vi "HFRR ADV v03.vi"() -> ()   [LabVIEW 2025] (continued)
                n448 = Concatenate Strings("FF ( V ); DP( mincron ) " ("character string"), "\r") -> (w782:string)
                n449 = local read "file count"() -> (w765:i32)
                n450 = local read "FILE 2"() -> (w770:string)
                n451 = local write "save dpt"(FALSE ("Hold 3")) -> ()
                n452 = Number To Decimal String(number=w765) -> (decimal integer string=w771:string)  [unwired: 1 in]
                n453 = Concatenate Strings(w770, w771) -> (w763:string)
                n454 = Concatenate Strings("C:\\LAB-IQ-NXT\\data" ("Substring"), w763) -> (w778:string)
                n455 = Concatenate Strings(w778, ".dpf" ("Substring")) -> (w776:string)
                n456 = Add(x=1, y=w765) -> (x+y=w766:i32)
                n457 = local write "file count"(w766) -> ()
                n458 = String To Path(string=w776) -> (path=w774:path)
                n459 = call <vilib>:"Write Characters To File.vi"("append to file? (new file:F)"=FALSE, "character string"=w782, "file path (dialog if empty)"=w774) -> ("new file path (Not A Path if cancelled)"=w779:path)  [unwired: 2 in]
                n460 = call <vilib>:"Write Characters To File.vi"("append to file? (new file:F)"=TRUE, "character string"=w769, "file path (dialog if empty)"=w779) -> ()  [unwired: 2 in, 1 out]
              }
            }
          }
          frame #5 {
            n461 = case shown="True" "Hold 4" {
              frame False {
              }
              frame True {
                n462 = File Dialog(6:"*.dpf" ("pattern"), 11:path "C:/LAB-IQ-NXT" ("start path")) -> (0:w789:errorcluster, 3:w804:path)  [unwired: 5 in, 2 out]
                n463 = Unbundle(w789) -> ()  [unwired: 3 out]
                n464 = call <vilib>:"Read Characters From File.vi"("file path (dialog if empty)"=w804) -> ("character string"=w794:string)  [unwired: 5 in, 3 out]
                n465 = Spreadsheet String To Array(delimiter (Tab)=";", format string="%S", spreadsheet string=w794, array type (2D Dbl)=string[][] []) -> (array=w798:string[][])
                n466 = for {
                  tunnel: w798 -> [w808] mode=indexing
                  tunnel: [w807] -> w799 mode=indexing
                  n467 = for {
                    tunnel: w808 -> [w810] mode=indexing
                    tunnel: [w809] -> w807 mode=indexing
                    n468 = call <vilib>:"Trim Whitespace.vi"("string"=w810) -> ("trimmed string"=w809:string)  [unwired: 1 in]
                  }
                }
                n469 = Fract/Exp String To Number(string=w799) -> (number=w801:dbl[][])  [unwired: 3 in, 1 out]
                n470 = Array Subset(array=w801, index (row)=1 ("index (col)")) -> (w803:dbl[][])  [unwired: 3 in]
                n471 = Index Array(array=w803, index (col) #1=0 ("disabled index (col)"), index (col) #2=1 ("disabled index (col)")) -> (element #1=w792:dbl[], element #2=w791:dbl[])  [unwired: 2 in]
                n472 = Build Array(w792, w791) -> (→"Waveform Graph":dbl[][])
              }
            }
          }
        }
      }
      frame Error {
        w826 = u16 0 items=["None", "XON/XOFF", "RTS/CTS", "XON/XOFF & RTS/CTS", "DTR/DSR", "XON/XOFF & DTR/DSR"] ("flow control (0:none)  2")
        w824 = u16 10 items=["1.0"=10, "1.5"=15, "2.0"=20] ("stop bits 2")
        w822 = u16 0 items=["None", "Odd", "Even", "Mark", "Space"] ("parity 2")
        w823 = u32 10000  # timeout (10sec)
        n473 = VISA Close(VISA resource name=w818, error in (no error)=w815) -> (error out=w819:errorcluster)
        n474 = local read "Com Port 1"() -> (w811:refnum<visa-resource-name>)
        n475 = call <vilib>:"Clear Errors.vi"("error in (no error)"=w819) -> ("error out"=w816:errorcluster)  [unwired: 5 in, 1 out]
        n476 = local write "Sps 3"(0.0 ("Sps 4")) -> ()
        n477 = call-poly "VISA Configure Serial Port"("VISA resource name"=w811, "timeout (10sec)"=w823, "baud rate (9600)"=u32 250000 ("baud rate  2"), "data bits (8)"=u16 8 ("data bits  2"), "parity (0:none)"=w822, "error in (no error)"=w816, "stop bits (10: 1 bit)"=w824, "flow control (0:none)"=w826) -> ("VISA resource name out"=w827:refnum<visa-resource-name>, "error out"=w828:errorcluster)  [unwired: 6 in]
        n478 = flat-sequence {
          tunnel: w827 -> [w830]
          tunnel: w828 -> [w829]
          tunnel: [w830] -> w820
          tunnel: [w829] -> w812
          frame #0 {
            n479 = Wait (ms)(milliseconds to wait=u32 50) -> ()  [unwired: 1 out]
          }
        }
        "Residual Uno" <- ""
        "Port 1 Error" <- w812
      }
    }
    n480 = local read "Port 1a"() -> (w473:bool)
    n481 = local read "Port 3"() -> (w474:bool)
    n482 = Or(x=w474, y=w473) -> (x .or. y?=w476:bool)
    n483 = case shown="False" w476 {
      frame False {
        w487 = FALSE ("Visible")
        n484 = property on="Port 1a" class="Bool (strict)"("Visible"=w487) -> ()  [unwired: 2 in, 2 out]
        n485 = property on="Port 3" class="Bool (strict)"("Visible"=w487) -> ()  [unwired: 2 in, 2 out]
      }
      frame True {
        w488 = TRUE ("Visible")
        n486 = property on="Port 1a" class="Bool (strict)"("Visible"=w488) -> ()  [unwired: 2 in, 2 out]
        n487 = property on="Port 3" class="Bool (strict)"("Visible"=w488) -> ()  [unwired: 2 in, 2 out]
      }
    }
    n488 = local read "EXIT"() -> (w478:bool)
    "Error Uno" <- w472
  }
  n489 = while {
    tunnel: w54 -> [_]
    tunnel: [w853] -> _
    tunnel: w23 -> [_]
    tunnel: ["EXIT"] -> w51
    i -> [w853]
    stop <- "EXIT" stop-if-true
    # "C:\\LAB-IQ-NXT\\Scar View.exe"
    n490 = local read "RUN"() -> (w851:bool)
    n491 = local read "EDIT 2"() -> (w838:bool)
    n492 = case shown="False" w851 {
      frame False {
        n493 = local read "stopT"() -> (w1724:bool)
        n494 = case shown="True" w1724 {
          frame False {
          }
          frame True {
            w1725 = FALSE
            n495 = local write "st enable"(w1725) -> ()
            n496 = local write "stopT"(w1725) -> ()
          }
        }
      }
      frame True {
        "stopT" <- TRUE
      }
    }
    n497 = case shown="True" w838 {
      frame False {
        n498 = local write "Password 2"("" ("Password")) -> ()
        n499 = property on="Password 2" class="Str"("Visible"=FALSE) -> ()  [unwired: 2 in, 2 out]
      }
      frame True {
        n500 = property on="Password 2" class="Str"("Visible"=TRUE) -> ()  [unwired: 2 in, 2 out]
        n501 = Equal?(x="Password 2", y="HFRR1234") -> (x = y?=w866:bool)
        n502 = case shown="True" w866 {
          tunnel: "Password 2" -> [w869 _]
          frame False {
            n503 = String Length(string=w869) -> (length=w870:i32)
            n504 = Greater Than 0?(x=w870) -> (x > 0?=w868:bool)
            n505 = case shown="False" w868 {
              frame False {
                n506 = property on="Password 2" class="Str"("Caption.Text"="Password (Advance Setting)") -> ()  [unwired: 2 in, 2 out]
              }
              frame True {
                n507 = property on="Password 2" class="Str"("Caption.Text"="Incorrect Password!") -> ()  [unwired: 2 in, 2 out]
              }
            }
          }
          frame True {
            n508 = local write "Password 2"("" ("Password")) -> ()
            n509 = local write "Main Tab"(T1."Advance" ("Main Tab")) -> ()
            n510 = local write "EDIT 2"(FALSE ("EDIT 2")) -> ()
          }
        }
      }
    }
    n511 = Wait (ms)(milliseconds to wait=u32 50) -> ()  [unwired: 1 out]
    n512 = case shown="True" "EDIT 3" {
      frame False {
      }
      frame True {
        n513 = local write "EDIT 3"(FALSE ("EDIT 3")) -> ()
        n514 = local write "Main Tab"(T1."About" ("Main Tab")) -> ()
      }
    }
    n515 = local read "Re-Initialise"() -> (w836:bool)
    n516 = case shown="True" w836 {
      frame False {
      }
      frame True {
        n517 = local write "Re-Initialise"(FALSE ("Re-Initialise")) -> ()
      }
    }
    n518 = case shown="\"ASTM D6079\", Default" "TEST STANDARD" {
      tunnel: [2.0 ("Set Temp") 0.0 ("Set Temp") 2.0 ("Set Temp") 0.0 ("Set Temp")] -> w839
      frame "ASTM D6079", Default {
        # "astm hide"
        n519 = local write "Set Hz"(50.0 ("Hz")) -> ()
        n520 = local write "Set Strk"(1.0 ("Set Strk")) -> ()
        n521 = local write "Set Rh"(53.0 ("Set Rh")) -> ()
        n522 = local write "Set Temp"(60.0 ("Set Temp")) -> ()
        n523 = local write "test time"(75.0 ("test time")) -> ()
        n524 = local write "NORMAL LOAD"(2.0 ("NORMAL LOAD")) -> ()
        "Test Standard" <- "ASTM D6079" ("Test Standard 2")
      }
      frame "ISO 12156" {
        n525 = local write "Set Hz"(50.0 ("Hz")) -> ()
        n526 = local write "Set Rh"(53.0 ("Set Rh")) -> ()
        n527 = local write "Set Strk"(1.0 ("Set Strk")) -> ()
        n528 = local write "test time"(75.0 ("test time")) -> ()
        n529 = local write "Set Temp"(60.0 ("Set Temp")) -> ()
        n530 = local write "NORMAL LOAD"(2.0 ("NORMAL LOAD")) -> ()
      }
      frame "CEC F-096-A-06" {
        n531 = local write "Set Strk"(1.0 ("Set Strk")) -> ()
        n532 = local write "Set Hz"(50.0 ("Hz")) -> ()
        n533 = local write "Set Rh"(53.0 ("Set Rh")) -> ()
        n534 = local write "Set Temp"(60.0 ("Set Temp")) -> ()
        n535 = local write "test time"(75.0 ("test time")) -> ()
        n536 = local write "NORMAL LOAD"(2.0 ("NORMAL LOAD")) -> ()
      }
      frame "Custom" {
      }
    }
    n537 = local read "OPEN 6"() -> (w835:bool)
    n538 = local read "service 3"() -> (w833:bool)
    n539 = Or(x=w835, y=w833) -> (x .or. y?=w834:bool)
    n540 = local read "RUN"() -> (w848:bool)
    n541 = case shown="True" w834 {
      selector: w834 -> [_ w858]
      frame False {
      }
      frame True {
        n542 = Not(x=w858) -> (.not. x?=w854:bool)
        n543 = local write "service 3"(w854) -> ()
        n544 = local write "OPEN 6"(w854) -> ()
        n545 = call <vilib>:"System Exec.vi"("wait until completion? (T)"=TRUE, "command line"="C:\\LAB-IQ-NXT\\Scar View.exe") -> ("error out"=→"error out 5":errorcluster)  [unwired: 6 in, 3 out]
      }
    }
    n546 = case shown="True" w848 {
      frame False {
      }
      frame True {
        n547 = local read "Main Tab"() -> (w1722:T1)
        n548 = case shown="\"Compare Files\"" w1722 {
          frame "Acquire", Default {
          }
          frame "Compare Files" {
            n549 = local write "Main Tab"(T1."Acquire" ("Main Tab")) -> ()
          }
          frame "About" {
          }
        }
      }
    }
    n550 = local read "Main Tab"() -> (w832:T1)
    n551 = case shown="\"Compare Files\"" w832 {
      tunnel: [T12."Acquire" ("Main Tab") T13."   COMPARE   FILES " ("Tab Control") T14."PRINT REPORT" ("Tab Control")] -> w846
      frame "Acquire", Default {
      }
      frame "Compare Files" {
      }
      frame "About" {
      }
    }
    n552 = property on="SetTemp" class="DigNum (strict)"("Disabled"=w839) -> ()  [unwired: 2 in, 2 out]
    n553 = case shown="0, Default" w846 {
      frame 0, Default {
        w1866 = 0.2 ("y")
        w1871 = 1.0 ("y")
        w1872 = 0.8 ("y")
        # "Elapsed time\ncof\nstroke\nAir temp\nTemp\nHumidity"
        n554 = case shown="True" "Save & Continue" {
          frame False {
          }
          frame True {
            "acq 2" <- TRUE ("acq 2")
          }
        }
        n555 = case shown="True" "Save & Continue" {
          frame False {
          }
          frame True {
            n556 = while {
              tunnel: "0123456789abcdefghijklmnopqrstuvwxyzABCDEFGHIJKLMNOPQRSTUVWXYZ" ("string 2") -> [w1990]
              shift-right: [w1988] -> w1983
              shift-left: "" -> [w1987]
              i -> [w1997]
              stop <- w1996 stop-if-true
              n557 = Random Number (0-1)() -> (number: 0 to 1=w1991:dbl)
              n558 = Multiply(x=w1991, y=62.0) -> (x*y=w1993:dbl)
              n559 = Decrement(x="Length") -> (x-1=w1986:i16)
              n560 = To Word Integer(number=w1993) -> (16bit integer=w1994:i16)
              n561 = String Subset(string=w1990, offset (0)=w1994, length (rest)=1 ("length (rest)")) -> (substring=w1989:string)
              n562 = Greater Or Equal?(x=w1997, y=w1986) -> (x >= y?=w1996:bool)
              n563 = Concatenate Strings(w1989, w1987) -> (w1988:string)
            }
            n564 = local write "UUID"(w1983) -> ()
          }
        }
        n565 = case shown="True" "Save & Continue" {
          frame False {
          }
          frame True {
            n566 = local read "Operator ID"() -> (w2273:string)
            n567 = local read "FILE"() -> (w2280:string)
            n568 = String Length(string=w2273) -> (length=w2274:i32)
            n569 = String Length(string=w2280) -> (length=w2278:i32)
            n570 = Greater?(x=w2274, y=0) -> (0:w2272:bool)
            n571 = Greater?(x=w2278, y=0) -> (0:w2277:bool)
            n572 = And(x=w2277, y=w2272) -> (x .and. y?=w2276:bool)
            n573 = case shown="True" w2276 {
              frame False {
                n574 = stacked-sequence {
                  frame #0 {
                    n575 = One Button Dialog(message="Please Enter a File Name and Operator ID to save data !", button name ("OK")="Ok") -> ()  [unwired: 1 out]
                  }
                  frame #1 {
                    n576 = local write "Save & Continue"(FALSE ("OK Button")) -> ()
                  }
                }
                n577 = local write "Save & Continue"(FALSE ("OK Button")) -> ()
              }
              frame True {
                n578 = stacked-sequence {
                  frame #0 {
                    (unwired) ")!" ("string")
                    (unwired) ")" ("string")
                    w2285 = dbl[] [] ("History Data")
                    w2289 = "\r"
                    # "C:\\WinDucom\\Data\\"
                    # "C:\\LAB-IQ-NXT\\data"
                    n579 = local read "Batch Ref Num :"() -> (w2287:string)
                    n580 = local read "NORMAL LOAD"() -> (w2306:dbl)
                    n581 = local read "Fuel Discription :"() -> (w2300:string)
                    n582 = Multiply(x=w2306, y=1.0) -> (x*y=w2305:dbl)
                    n583 = Number To Fractional String(number=w2305, width (-)=i16 5, precision (6)=i16 2) -> (F-format string=w2314:string)  [unwired: 1 in]
                    n584 = Concatenate Strings(w2300) -> (w2301:string)
                    n585 = local read "Remarks :"() -> (w2299:string)
                    n586 = property on="Electronic contact resistance ( % )" class="WFChart (strict)"("History Data"=w2285) -> ()  [unwired: 2 in, 2 out]
                    n587 = Get Date/Time String(date format (0)=enum16{"short", "long", "abbreviated"}."short") -> (date string=w2325:string, time string=w2322:string)  [unwired: 2 in]
                    n588 = property on="Coefficient of Friction" class="WFChart (strict)"("History Data"=w2285) -> ()  [unwired: 2 in, 2 out]
                    n589 = property on="Frictional Force ( N )" class="WFChart (strict)"("History Data"=w2285) -> ()  [unwired: 2 in, 2 out]
                    n590 = Concatenate Strings(w2287) -> (w2286:string)
                    n591 = Concatenate Strings(w2299, "," ("string")) -> (w2298:string)
                    n592 = Concatenate Strings("Load :- " ("Substring"), w2314, " N ," ("Substring")) -> (w2313:string)
                    n593 = local read "String 41"() -> (w2291:string)
                    n594 = local read "FILE"() -> (w2333:string)
                    n595 = Concatenate Strings("(" ("Substring"), w2325, ")" ("Substring"), w2322) -> (w2293:string)
                    "concatenated string" <- w2293
                    n596 = Concatenate Strings("C:\\LAB-IQ-NXT\\data\\" ("string"), w2333) -> (w2332:string)
                    n597 = Concatenate Strings("tested by") -> (w2295:string)
                    n598 = Concatenate Strings(w2332, ".duf" ("Substring")) -> (w2329:string)
                    n599 = Concatenate Strings(w2332, ".dgf" ("Substring")) -> (w2328:string)
                    n600 = String To Path(string=w2328) -> (path=w2326:path)
                    n601 = String To Path(string=w2329) -> (path=w2303:path)
                    n602 = Concatenate Strings(w2291, w2289, "Fuel Discription :-" ("Substring"), w2301, w2289, w2313, w2289, "Batch Ref Num :-" ("Substring"), w2286, w2289, " Remarks :- " ("Substring"), w2298, w2289, " Date :- " ("Substring"), w2293, w2289, "Tested By :-" ("Substring"), w2295) -> (w2307:string)
                    "REMARKS" <- w2307
                    n603 = local write "clk"(0.0 ("clk")) -> ()
                    n604 = local write "speedop"(0.0 ("PIDclk 2")) -> ()
                    n605 = Concatenate Strings("  TIME;      COF;       STROKE;     AIR TEMP;  TEMP;  HUMIDITY;  ECR; PID-OUT; FREQUENCY" ("Substring"), "\r") -> (w2309:string)
                    n606 = call <vilib>:"Write Characters To File.vi"("append to file? (new file:F)"=FALSE, "character string"=w2309, "file path (dialog if empty)"=w2326) -> ()  [unwired: 2 in, 1 out]
                    n607 = call <vilib>:"Write Characters To File.vi"("append to file? (new file:F)"=FALSE, "character string"=w2307, "file path (dialog if empty)"=w2303) -> ()  [unwired: 2 in, 1 out]
                  }
                  frame #1 {
                    n608 = local write "autostrtflg"(TRUE ("autostrtflg")) -> ()
                    n609 = local write "Save & Continue"(FALSE ("OK")) -> ()
                    n610 = local write "STOP 3"(FALSE ("STOP")) -> ()
                    n611 = One Button Dialog(message="Please ensure sample is mounted properly and machine is ready in all aspects for testing !", button name ("OK")="Ok") -> ()  [unwired: 1 out]
                    n612 = property on="Save & Continue" class="Bool (strict)"("Visible"=FALSE ("OK")) -> ()  [unwired: 2 in, 2 out]
                    n613 = property on="STOP 3" class="Bool (strict)"("Visible"=TRUE) -> ()  [unwired: 2 in, 2 out]
                    n614 = Get Date/Time In Seconds() -> (seconds since 1Jan1904=w2338:timestamp)
                    n615 = local write "Cycles elapsed"(0 ("Cycles elapsed")) -> ()
                    n616 = To Double Precision Float(number=w2338) -> (double precision float=w2337:dbl)
                    n617 = local write "cyclecount"(0 ("cyclecount")) -> ()
                    n618 = local write "acq timer"(w2337) -> ()
                    n619 = local write "Save"(FALSE ("Save")) -> ()
                  }
                }
              }
            }
          }
        }
        n620 = case shown="True" "Case Constant\n(See Context Help) 15" {
          frame False {
          }
          frame True {
            n621 = local read "zflag 2"() -> (w1898:dbl)
            n622 = local read "yflag"() -> (w1900:dbl)
            n623 = Equal?(x=w1898, y=3.0 ("tflag")) -> (x = y?=w1901:bool)
            n624 = Equal?(x=w1900, y=2.0 ("tflag")) -> (x = y?=w1902:bool)
            n625 = And(x=w1902, y=w1901) -> (x .and. y?=w1896:bool)
            n626 = case shown="True" w1896 {
              frame False {
              }
              frame True {
                w1927 = 0.0 ("zflag")
                n627 = local read "SEN.RUN HRS"() -> (w1913:dbl)
                n628 = local read "SENSOR TIME"() -> (w1911:dbl)
                n629 = local read "Total No. of Tests"() -> (w1914:dbl)
                n630 = Delete(path (use dialog)=path "C:/LAB-IQ-NXT/WO 2449 TRH.sig" ("file path (dialog if empty)")) -> (deleted path=w1921:path)  [unwired: 4 in, 2 out]
                n631 = Add(x=w1911, y=w1913) -> (x+y=w1912:dbl)
                "SEN.RUN HRS" <- w1912
                n632 = Number To Decimal String(number=w1912) -> (decimal integer string=w1918:string)  [unwired: 1 in]
                n633 = call <vilib>:"compatOverwrite.vi"("overwrite (F)"=TRUE) -> ("overwrite?"=w1907:T17)
                n634 = Delete(path (use dialog)=path "C:/LAB-IQ-NXT/WO 2449 TT.sig" ("file path (dialog if empty)")) -> (deleted path=w1926:path)  [unwired: 4 in, 2 out]
                n635 = Open/Create/Replace File(file path (use dialog)=w1921, operation (0:open)=w1907) -> (refnum out=w1908:refnum<file>, error out=w1909:errorcluster)  [unwired: 4 in, 1 out]
                n636 = Number To Decimal String(number=w1914) -> (decimal integer string=w1922:string)  [unwired: 1 in]
                n637 = Deny Access(4:w1909, 6:T15."deny none" ("deny mode (2)"), 7:w1908) -> (3:w1917:refnum<file>)  [unwired: 1 out]
                n638 = call <vilib>:"compatOverwrite.vi"("overwrite (F)"=TRUE) -> ("overwrite?"=w1903:T17)
                n639 = Write to Binary File(file (use dialog)=w1917, data=w1918, 5:FALSE ("prepend array or string size? (T)")) -> ()  [unwired: 3 in, 3 out]
                n640 = Open/Create/Replace File(file path (use dialog)=w1926, operation (0:open)=w1903) -> (refnum out=w1904:refnum<file>, error out=w1905:errorcluster)  [unwired: 4 in, 1 out]
                n641 = Deny Access(4:w1905, 6:T15."deny none" ("deny mode (2)"), 7:w1904) -> (3:w1925:refnum<file>)  [unwired: 1 out]
                n642 = local write "zflag"(w1927) -> ()
                n643 = local write "zflag 2"(w1927) -> ()
                n644 = Write to Binary File(file (use dialog)=w1925, data=w1922, 5:FALSE ("prepend array or string size? (T)")) -> ()  [unwired: 3 in, 3 out]
              }
            }
          }
        }
        n645 = case shown="True" "STOP 3" {
          frame False {
          }
          frame True {
            w2265 = "" ("Sample ID :")
            (unwired) FALSE ("Visible")
            n646 = local write "Save & Continue"(FALSE ("OK Button")) -> ()
            n647 = local write "STOP 3"(FALSE ("STOP")) -> ()
            n648 = local write "clk"(0.0 ("clk")) -> ()
            n649 = local write "RUN"(FALSE ("OK Button 2")) -> ()
            n650 = property on="Save & Continue" class="Bool (strict)"("Visible"=TRUE) -> ()  [unwired: 2 in, 2 out]
            n651 = property on="STOP 3" class="Bool (strict)"("Visible"=FALSE) -> ()  [unwired: 2 in, 2 out]
            n652 = property on="STOP 2" class="Bool (strict)"("Disabled"=u8 0) -> ()  [unwired: 2 in, 2 out]
            n653 = local write "Fuel Discription :"(w2265) -> ()
            n654 = local write "Remarks :"(w2265) -> ()
            n655 = local write "tested by"(w2265) -> ()
            n656 = local write "FILE"(w2265) -> ()
            n657 = local write "Batch Ref Num :"(w2265) -> ()
          }
        }
        n658 = local read "AIR TEMP"() -> (w1838:dbl)
        n659 = local read "run replace"() -> (w1878:bool)
        n660 = Greater Or Equal?(x=w1838, y=15.0) -> (x >= y?=w1839:bool)
        "powstat" <- w1839
        n661 = local read "acq 2"() -> (w1877:bool)
        n662 = And(x=w1877, y=w1878) -> (x .and. y?=w1876:bool)
        n663 = local read "run replace"() -> (w1879:bool)
        n664 = case shown="True" w1876 {
          frame False {
            n665 = local write "tfalg"(0.0 ("tfalg")) -> ()
          }
          frame True {
            n666 = local read "tfalg"() -> (w1974:dbl)
            n667 = Equal?(x=w1974, y=0.0) -> (x = y?=w1975:bool)
            n668 = case shown="True" w1975 {
              frame False {
              }
              frame True {
                n669 = local read "Total No. of Tests"() -> (w1978:dbl)
                n670 = Increment(x=w1978) -> (x+1=w1977:dbl)
                n671 = local write "Total No. of Tests"(w1977) -> ()
                n672 = local write "tfalg"(1.0 ("tfalg")) -> ()
                n673 = local write "acq 2"(FALSE ("acq 2")) -> ()
                n674 = Wait (ms)(milliseconds to wait=u32 200) -> ()  [unwired: 1 out]
              }
            }
          }
        }
        n675 = case shown="False" w1879 {
          frame False {
            n676 = local read "zflag"() -> (→"zflag 2":dbl)
            n677 = local write "FLAG 4"(0.0 ("FLAG")) -> ()
            n678 = local write "yflag"(2.0 ("tflag")) -> ()
          }
          frame True {
            n679 = local write "zflag"(3.0 ("zflag")) -> ()
            n680 = local write "yflag"(1.0 ("tflag")) -> ()
          }
        }
        n681 = property on="STOP 3" class="Bool (strict)"() -> ("Visible"=w1881:bool)  [unwired: 2 in, 2 out]
        n682 = case shown="True" w1881 {
          tunnel: [FALSE ("Visible") TRUE ("Visible")] -> w1891
          frame False {
          }
          frame True {
          }
        }
        n683 = property on="RUN" class="Bool (strict)"("Visible"=w1891) -> ()  [unwired: 2 in, 2 out]
        n684 = property on="Save & Continue" class="Bool (strict)"() -> ("Visible"=w1894:bool)  [unwired: 2 in, 2 out]
        n685 = local read "RUN"() -> (w1875:bool)
        n686 = case shown="True" w1875 {
          frame False {
            n687 = local read "Rt 3"() -> (w1956:bool)
            n688 = case shown="True" w1956 {
              frame False {
              }
              frame True {
                n689 = local write "Json End Flg"(TRUE ("Upld AR 2")) -> ()
                n690 = local write "Rt 3"(FALSE ("Rt 3")) -> ()
              }
            }
            "Rt" <- TRUE ("Rt")
            "Rt 2" <- FALSE ("Rt")
          }
          frame True {
            n691 = local read "Rt"() -> (w1963:bool)
            n692 = case shown="True" w1963 {
              frame False {
              }
              frame True {
                w1964 = TRUE ("Upld AR 2")
                n693 = local write "Rt"(FALSE ("Rt")) -> ()
                n694 = local write "Upld AR"(w1964) -> ()
                n695 = local write "Json St Flg"(w1964) -> ()
              }
            }
            n696 = local write "Rt 2"(TRUE ("Rt 2")) -> ()
            "Rt 3" <- TRUE ("Rt 3")
          }
        }
        n697 = Not(x=w1894) -> (.not. x?=w1893:bool)
        n698 = case shown="True" w1875 {
          frame False {
            n699 = local write "run replace"(FALSE ("run replace")) -> ()
          }
          frame True {
            "run replace" <- TRUE ("run replace")
          }
        }
        n700 = And(x=w1893, y=w1881) -> (x .and. y?=w1890:bool)
        "Test Status 2" <- w1890
        n701 = case shown="True" w1890 {
          tunnel: w1839 -> [_ w2029]
          frame False {
            w2027 = 0.0 ("output")
            n702 = local write "Frequency ( Hz )"(w2027) -> ()
            n703 = local write "PID-out"(w2027) -> ()
            n704 = local write "Heater Button"(FALSE ("Heater Button")) -> ()
          }
          frame True {
            n705 = case shown="False" w2029 {
              frame False {
                n706 = stacked-sequence {
                  frame #0 {
                    n707 = local write "RUN"(FALSE ("OK Button 2")) -> ()
                  }
                  frame #1 {
                    n708 = property on="RUN" class="Bool (strict)"("Visible"=FALSE) -> ()  [unwired: 2 in, 2 out]
                  }
                }
              }
              frame True {
              }
            }
            n709 = stacked-sequence {
              frame #0 {
                n710 = case shown="True" "RUN" {
                  tunnel: [w2056 w2064] -> w2033
                  frame False {
                    w2056 = 0.0
                    n711 = local write "Reinit PID"(TRUE) -> ()
                    n712 = property on="Stroke 2" class="DigNum (strict)"("Visible"=FALSE) -> ()  [unwired: 2 in, 2 out]
                    n713 = property on="Stroke" class="DigNum (strict)"("Visible"=TRUE) -> ()  [unwired: 2 in, 2 out]
                    n714 = local write "String 14"("Test will autostart once parameters reach the set value." ("String 14")) -> ()
                    n715 = local write "Old Pid Val"(w2056) -> ()
                  }
                  frame True {
                    n716 = local read "PID Ref"() -> (w2075:bool)
                    n717 = property on="STOP 2" class="Bool (strict)"("Disabled"=u8 2) -> ()  [unwired: 2 in, 2 out]
                    n718 = case shown="True" w2075 {
                      tunnel: [w2076 w2092] -> w2074
                      frame False {
                        n719 = local read "Old Pid Val"() -> (w2076:dbl)
                      }
                      frame True {
                        n720 = local read "Set Hz"() -> (w2085:dbl)
                        n721 = Add(x=w2085, y=-10.0 ("Offset")) -> (x+y=w2103:dbl)
                        n722 = local read "Frequency"() -> (w2096:dbl)
                        n723 = Add(x=w2085, y=-10.0) -> (x+y=w2095:dbl)
                        n724 = Add(x=w2085, y=10.0) -> (x+y=w2094:dbl)
                        n725 = Multiply(x=w2103, y=0.1 ("Gain")) -> (x*y=w2082:dbl)
                        n726 = Add(x=w2082, y=1.5) -> (x+y=w2080:dbl)
                        n727 = local read "SPEED OUT:"() -> (w2104:dbl)
                        n728 = In Range and Coerce(upper limit=w2094, x=w2096, lower limit=w2095) -> (coerced(x)=w2084:dbl)  [unwired: 1 out]
                        n729 = Multiply(x=w2080, y=w2104) -> (x*y=w2079:dbl)
                        n730 = Multiply(x=w2079, y=0.8) -> (x*y=w2078:dbl)
                        n731 = local read "Elapsed time"() -> (w2089:dbl)
                        n732 = Or(x="Reinit PID", y="Reinit PID") -> (x .or. y?=w2093:bool)
                        n733 = call-poly <vilib>:"PID.vi"("reinitialize? (F)"=w2093, "output range"=cluster{"output high":dbl, "output low":dbl} {"output high"=1.0, "output low"=-1.0}, "PID gains"=T7 {"proportional gain (Kc)"=0.0005, "integral time (Ti, min)"=0.001, "derivative time (Td, min)"=0.0} ("Motor PID"), "process variable"=w2084, "setpoint"=w2085) -> ("output"=w2083:dbl)  [unwired: 5 in, 1 out]
                        n734 = Greater?(x=w2089, y=0.05) -> (0:w2088:bool)
                        n735 = case shown="True" w2088 {
                          tunnel: w2083 -> [_ w2106]
                          tunnel: [0.0 ("output") w2106] -> w2086
                          frame False {
                          }
                          frame True {
                            n736 = local write "Reinit PID"(FALSE ("Reinit PID")) -> ()
                          }
                        }
                        n737 = Add(x=w2078, y=w2086) -> (x+y=w2091:dbl)
                        n738 = flat-sequence {
                          tunnel: [w2109] -> w2092
                          tunnel: w2091 -> [w2109]
                          frame #0 {
                            n739 = local write "PID Ref"(FALSE ("PID Ref")) -> ()
                          }
                        }
                      }
                    }
                    "Old Pid Val" <- w2074
                    n740 = local read "Set Hz"() -> (w2071:dbl)
                    n741 = local read "Freq"() -> (w2063:dbl)
                    n742 = call <vilib>:"Uniform White Noise Waveform.vi"() -> ("signal out"=w2070:waveform(dbl))  [unwired: 10 in, 1 out]
                    n743 = property on="RUN" class="Bool (strict)"("Visible"=TRUE) -> ()  [unwired: 2 in, 2 out]
                    n744 = Add(x=w2071, y=w2070) -> (x+y=w2069:waveform(dbl))
                    n745 = property on="Stroke 2" class="DigNum (strict)"("Visible"=TRUE) -> ()  [unwired: 2 in, 2 out]
                    n746 = property on="Stroke" class="DigNum (strict)"("Visible"=FALSE) -> ()  [unwired: 2 in, 2 out]
                    n747 = Multiply(x=w2069, y=ext 0.1) -> (x*y=w2065:waveform(ext))
                    n748 = Multiply(x=w2063, y=0.9) -> (x*y=w2066:dbl)
                    n749 = local write "String 14"(" Running....." ("String 14")) -> ()
                    n750 = Add(x=w2065, y=w2066) -> (x+y=w2064:waveform(ext))
                  }
                }
                n751 = Not(x="Engage") -> (.not. x?=w2037:bool)
                n752 = call "Elapsed Time"("Time Target (s)"="Countdown", "Reset"=w2037) -> ("Elapsed Time (s)"=w2042:dbl, "Time has Elapsed"=w2040:bool)  [unwired: 10 in, 6 out]
                "Countdown 2" <- w2042
                n753 = Subtract(x=w2042, y=2.0) -> (x-y=w2045:dbl)
                n754 = Less?(x=w2045, y="Countdown") -> (x < y?=w2043:bool)
                n755 = And(x=w2043, y=w2040) -> (x .and. y?=w2039:bool)
                n756 = case shown="True" w2039 {
                  frame False {
                  }
                  frame True {
                    n757 = local read "Humidity ( Rh )"() -> (→"Rh Before":dbl)
                    n758 = local write "RUN"(TRUE ("RUN")) -> ()
                    n759 = local write "Engage"(FALSE ("Engage")) -> ()
                    n760 = property on="gRh" class="WFChart (strict)"("History Data"=dbl[] []) -> ()  [unwired: 2 in, 2 out]
                  }
                }
                n761 = local read "clk"() -> (w2050:dbl)
                n762 = local read "Save"() -> (w2046:bool)
                n763 = Equal?(x=w2050, y=0.0) -> (x = y?=w2047:bool)
                n764 = And(x=w2047, y=w2046) -> (x .and. y?=w2048:bool)
                n765 = case shown="True" w2048 {
                  frame False {
                  }
                  frame True {
                    n766 = Get Date/Time In Seconds() -> (seconds since 1Jan1904=w2112:timestamp)
                    n767 = To Double Precision Float(number=w2112) -> (double precision float=w2110:dbl)
                    n768 = local write "act save time"(w2110) -> ()
                    n769 = local write "acq timer"(w2110) -> ()
                    n770 = local write "clk"(10.0 ("clk")) -> ()
                  }
                }
                n771 = local read "Test \nStatus"() -> (w2035:bool)
                n772 = Select(t=w2033, s=w2035, f=0.0) -> (s? t:f=w2034:dbl)
                n773 = local write "Frequency ( Hz )"(w2034) -> ()
                n774 = local write "Freq"(w2034) -> ()
              }
              frame #1 {
                w2135 = 1000000.0 ("x")
                # "Elapsed time\ncof\nstroke\nAir temp\nTemp\nHumidity"
                # "acq timer\n\nact save time"
                # "convert to microseconds"
                n775 = local read "COUNT"() -> (w2118:i32)
                n776 = Greater Or Equal?(x=w2118, y=250) -> (x >= y?=w2117:bool)
                n777 = case shown="True" w2117 {
                  frame False {
                    n778 = local read "COUNT"() -> (w2139:i32)
                    n779 = Increment(x=w2139) -> (x+1=w2140:i32)
                    n780 = local write "COUNT"(w2140) -> ()
                  }
                  frame True {
                    n781 = local write "COUNT"(0 ("COUNT")) -> ()
                  }
                }
                n782 = local read "Samplingtime 2"() -> (w2116:dbl)
                n783 = local read "act save time"() -> (w2133:dbl)
                n784 = Get Date/Time In Seconds() -> (seconds since 1Jan1904=w2138:timestamp)
                n785 = To Double Precision Float(number=w2138) -> (double precision float=w2127:dbl)
                n786 = local read "acq timer"() -> (w2137:dbl)
                n787 = Add(x=w2133, y=w2116) -> (x+y=w2132:dbl)
                n788 = Greater Or Equal?(x=w2127, y=w2132) -> (x >= y?=w2115:bool)
                n789 = Subtract(x=w2127, y=w2137) -> (x-y=w2129:dbl)
                n790 = local read "Rate"() -> (w2131:dbl)
                n791 = Divide(x=w2135, y=w2131) -> (x/y=w2136:dbl)
                n792 = Divide(x=w2136, y=w2135) -> (x/y=w2134:dbl)
                n793 = local read "Save"() -> (w2130:bool)
                n794 = And(x=w2115, y=w2130) -> (x .and. y?=w2128:bool)
                n795 = case shown="True" w2128 {
                  tunnel: w2127 -> [_ w2210]
                  tunnel: [FALSE ("Boolean 2") TRUE ("Boolean 2")] -> _
                  frame False {
                  }
                  frame True {
                    w2178 = ";" ("Substring")
                    # "Pid out/\nFreq response value"
                    n796 = local write "act save time"(w2210) -> ()
                    n797 = local read "Set Strk"() -> (w2177:dbl)
                    n798 = local read "Stroke"() -> (w2167:dbl)
                    n799 = local read "FF 2"() -> (w2163:dbl)
                    "Frictional Force ( N )" <- w2163
                    n800 = Subtract(x=w2167, y=w2177) -> (x-y=w2174:dbl)
                    n801 = local read "TEMP"() -> (w2164:dbl)
                    "Temp" <- w2164
                    n802 = local write "FF 3"(w2163) -> ()
                    n803 = local read "ecr"() -> (w2162:dbl)
                    "ecr 2" <- w2162
                    n804 = Multiply(x=w2174, y=0.05) -> (x*y=w2176:dbl)
                    n805 = local read "Humidity ( Rh )"() -> (w2185:dbl)
                    "gRh" <- w2185
                    n806 = local read "Frequency ( Hz )"() -> (w2170:dbl)
                    n807 = local write "ecr 3"(w2162) -> ()
                    n808 = local read "COF 2"() -> (w2165:dbl)
                    "cof" <- w2165
                    "Coefficient of Friction" <- w2165
                    n809 = Add(x=w2176, y=w2177) -> (x+y=w2168:dbl)
                    "Stroke Ln" <- w2168
                    "Stroke 2" <- w2168
                    "Disp" <- w2168
                    n810 = local write "Temperature ( Deg C )"(w2164) -> ()
                    n811 = local read "Elapsed time"() -> (w2203:dbl)
                    n812 = local write "COF 3"(w2165) -> ()
                    n813 = local read "AIR TEMP"() -> (w2166:dbl)
                    n814 = local write "Electronic contact resistance ( % )"(w2162) -> ()
                    n815 = local read "PID-out"() -> (w2173:dbl)
                    n816 = local read "FILE"() -> (w2211:string)
                    n817 = Number To Fractional String(number=w2165, width (-)=i16 9 ("precision (6)"), precision (6)=i16 6) -> (F-format string=w2204:string)  [unwired: 1 in]
                    n818 = Number To Fractional String(number=w2168, width (-)=i16 9 ("precision (6)"), precision (6)=i16 6) -> (F-format string=w2196:string)  [unwired: 1 in]
                    n819 = Number To Fractional String(number=w2166, width (-)=i16 9 ("precision (6)"), precision (6)=i16 3) -> (F-format string=w2195:string)  [unwired: 1 in]
                    n820 = Number To Fractional String(number=w2164, width (-)=i16 9 ("precision (6)"), precision (6)=i16 3) -> (F-format string=w2192:string)  [unwired: 1 in]
                    n821 = Number To Fractional String(number=w2185, width (-)=i16 9 ("precision (6)"), precision (6)=i16 3) -> (F-format string=w2189:string)  [unwired: 1 in]
                    n822 = Number To Fractional String(number=w2162, width (-)=i16 9 ("precision (6)"), precision (6)=i16 3) -> (F-format string=w2184:string)  [unwired: 1 in]
                    n823 = Number To Fractional String(number=w2173, width (-)=i16 9 ("precision (6)"), precision (6)=i16 3) -> (F-format string=w2179:string)  [unwired: 1 in]
                    n824 = Number To Fractional String(number=w2170, width (-)=i16 9 ("precision (6)"), precision (6)=i16 3) -> (F-format string=w2169:string)  [unwired: 1 in]
                    n825 = Number To Fractional String(number=w2203, width (-)=i16 14 ("precision (6)"), precision (6)=i16 3) -> (F-format string=w2205:string)  [unwired: 1 in]
                    n826 = Concatenate Strings("C:\\LAB-IQ-NXT\\Data\\" ("string"), w2211, ".dgf" ("Substring")) -> (w2213:string)
                    n827 = String To Path(string=w2213) -> (path=w2212:path)
                    n828 = Concatenate Strings(w2205, w2178, w2204, w2178, w2196, w2178, w2195, w2178, w2192, w2178, w2189, w2178, w2184, w2178, w2179, w2178, w2169, "\r") -> (w2202:string)
                    n829 = call <vilib>:"Write Characters To File.vi"("append to file? (new file:F)"=TRUE, "character string"=w2202, "file path (dialog if empty)"=w2212) -> ()  [unwired: 2 in, 1 out]
                    "refresh flag" <- TRUE ("refresh flag")
                  }
                }
                n830 = local read "COUNT"() -> (w2120:i32)
                n831 = Multiply(x=w2134, y=w2120) -> (x*y=w2126:dbl)
                n832 = Add(x=w2129, y=w2126) -> (x+y=w2113:dbl)
                "Elapsed time 3" <- w2113
                n833 = local read "Test \nStatus"() -> (w2114:bool)
                n834 = local read "clk"() -> (w2121:dbl)
                n835 = Equal?(x=w2121, y=10.0) -> (x = y?=w2123:bool)
                n836 = Divide(x=w2113, y=60.0) -> (x/y=w2124:dbl)
                n837 = case shown="True" w2114 {
                  tunnel: w2124 -> [_ w2146]
                  tunnel: w2129 -> [_ w2154]
                  tunnel: [0.0 w2150] -> _
                  tunnel: w2123 -> [_ w2149]
                  tunnel: [0.0 w2148] -> _
                  tunnel: w2113 -> [_ w2148]
                  tunnel: w2127 -> [w2142 _]
                  frame False {
                    n838 = local write "acq timer"(w2142) -> ()
                  }
                  frame True {
                    n839 = local read "Set Hz"() -> (w2151:dbl)
                    n840 = local write "Elapsed time"(w2146) -> ()
                    n841 = local read "test time"() -> (w2147:dbl)
                    n842 = Multiply(x=w2154, y=w2151) -> (x*y=w2153:dbl)
                    n843 = case shown="False" w2149 {
                      tunnel: w2153 -> [w2155 _]
                      tunnel: [w2155 1.0] -> w2150
                      frame False {
                        n844 = local write "Cycles elapsed"(w2155) -> ()
                      }
                      frame True {
                      }
                    }
                    n845 = Subtract(x=w2147, y=w2146) -> (x-y=w2145:dbl)
                    "time" <- w2145
                    n846 = Greater?(x=w2146, y=w2147) -> (0:w2152:bool)
                    n847 = case shown="True" w2152 {
                      frame False {
                      }
                      frame True {
                        n848 = local read "Humidity ( Rh )"() -> (→"Rh After":dbl)
                        n849 = property on="STOP 2" class="Bool (strict)"("Disabled"=u8 0) -> ()  [unwired: 2 in, 2 out]
                        n850 = local write "RUN"(FALSE ("OK Button 2")) -> ()
                        n851 = local write "STOP 3"(TRUE ("STOP")) -> ()
                      }
                    }
                    n852 = local write "Time Remaining"(w2145) -> ()
                  }
                }
              }
              frame #2 {
                n853 = case shown="True" "Heater Button" {
                  tunnel: [0.0 ("output") w2237] -> w2216
                  frame False {
                    w2218 = TRUE ("tmpchk")
                    n854 = local write "tmpchk"(w2218) -> ()
                    n855 = local write "Reset 4"(w2218) -> ()
                    n856 = local read "TEMP"() -> (w2219:dbl)
                    n857 = local write "Temp ini"(w2219) -> ()
                    n858 = local write "reinit"(TRUE ("reinit")) -> ()
                  }
                  frame True {
                    # "Logic to turn off\nthe heater when \ntemp is not rising.\nTime - 60 sec\nDelta t- 5°c"
                    n859 = local read "Set Temp"() -> (w2234:dbl)
                    n860 = local read "Temp ini"() -> (w2225:dbl)
                    n861 = local read "TEMP"() -> (w2228:dbl)
                    n862 = Add(x=w2234, y=0.5) -> (x+y=w2232:dbl)
                    n863 = Less?(x=w2225, y=53.0) -> (x < y?=w2223:bool)
                    n864 = Greater Or Equal?(x=w2228, y=w2232) -> ()  [unwired: 1 out]
                    n865 = And(x="tmpchk", y=w2223) -> (x .and. y?=w2226:bool)
                    n866 = case shown="True" w2226 {
                      frame False {
                      }
                      frame True {
                        n867 = call "Elapsed Time8"("Time Target (s)"=300.0, "Reset"="Reset 4") -> ("Time has Elapsed"=w2242:bool)  [unwired: 10 in, 7 out]
                        n868 = flat-sequence {
                          tunnel: w2242 -> [_]
                          frame #0 {
                            n869 = local write "Reset 4"(FALSE ("Reset 4")) -> ()
                          }
                        }
                        n870 = case shown="True" w2242 {
                          frame False {
                          }
                          frame True {
                            n871 = local read "Temp ini"() -> (w2249:dbl)
                            n872 = local read "TEMP"() -> (w2250:dbl)
                            n873 = Add(x=w2249, y=5.0) -> (x+y=w2247:dbl)
                            n874 = Greater?(x=w2250, y=w2247) -> (0:w2248:bool)
                            n875 = case shown="False" w2248 {
                              frame False {
                                n876 = local write "Heater Button"(FALSE ("Heater Button")) -> ()
                              }
                              frame True {
                                n877 = local write "tmpchk"(FALSE ("tmpchk")) -> ()
                              }
                            }
                          }
                        }
                      }
                    }
                    n878 = call-poly <vilib>:"PID.vi"("reinitialize? (F)"="reinit", "output range"="output range", "dt (s)"=-1.0, "PID gains"="Temp PID gains", "process variable"=w2228, "setpoint"=w2234) -> ("output"=w2231:dbl)  [unwired: 4 in, 1 out]
                    n879 = Select(t=0.0, s=FALSE, f=w2231) -> (s? t:f=w2230:dbl)
                    "PID output" <- w2230
                    n880 = Subtract(x=w2234, y=w2228) -> (x-y=w2236:dbl)
                    n881 = flat-sequence {
                      tunnel: w2230 -> [w2253]
                      tunnel: [w2253] -> w2237
                      frame #0 {
                        n882 = local write "reinit"(FALSE ("reinit")) -> ()
                      }
                    }
                    n883 = Bundle(w2236, "output"=w2230, "TEMP"=w2228) -> (→"gTEMP 3":cluster{dbl, "output":dbl, "TEMP":dbl})  [unwired: 1 in]
                  }
                }
                "PID-out" <- w2216
              }
              frame #3 {
                n884 = local read "TEMP"() -> (w2255:dbl)
                n885 = Greater Or Equal?(x=w2255, y="Set Temp 2") -> (x >= y?=w2260:bool)
                n886 = case shown="True" w2260 {
                  tunnel: [FALSE TRUE] -> w2258
                  frame False {
                  }
                  frame True {
                  }
                }
                "Status 13" <- w2258
                n887 = And(x=w2258, y="trip1 8") -> (x .and. y?=w2257:bool)
                n888 = case shown="True" w2257 {
                  frame False {
                  }
                  frame True {
                    w2261 = FALSE ("OK Button 2")
                    n889 = local write "Heater Button"(w2261) -> ()
                    n890 = local write "RUN"(w2261) -> ()
                  }
                }
              }
            }
          }
        }
        n891 = stacked-sequence {
          frame #0 {
            n892 = case shown="True" "RST FF" {
              frame False {
              }
              frame True {
                w2001 = 0.0 ("X Scale.Range:Maximum")
                n893 = property on="Frictional Force ( N )" class="WFChart (strict)"("XScale.Maximum"=600.0 ("X Scale.Range:Maximum"), "XScale.Minimum"=w2001, "YScale.Maximum"=10.0 ("Y Scale.Range:Maximum"), "YScale.Minimum"=w2001) -> ()  [unwired: 2 in, 2 out]
              }
            }
          }
          frame #1 {
            n894 = case shown="True" "RST TEMP" {
              frame False {
              }
              frame True {
                n895 = property on="Temperature ( Deg C )" class="WFChart (strict)"("XScale.Minimum"=0.0 ("X Scale.Range:Minimum"), "XScale.Maximum"=600.0 ("X Scale.Range:Maximum"), "YScale.Minimum"=0.0 ("Y Scale.Range:Minimum"), "YScale.Maximum"=100.0 ("Y Scale.Range:Maximum")) -> ()  [unwired: 2 in, 2 out]
              }
            }
          }
          frame #2 {
            n896 = case shown="True" "RSTCOF" {
              frame False {
              }
              frame True {
                n897 = property on="Coefficient of Friction" class="WFChart (strict)"("XScale.Minimum"=0.0 ("X Scale.Range:Minimum"), "XScale.Maximum"=600.0 ("X Scale.Range:Maximum"), "YScale.Maximum"=1.0 ("X Scale.Range:Minimum"), "YScale.Minimum"=0.0 ("X Scale.Range:Minimum")) -> ()  [unwired: 2 in, 2 out]
              }
            }
          }
          frame #3 {
            n898 = case shown="True" "RSTCOF 2" {
              frame False {
              }
              frame True {
                (unwired) 100.0 ("Y Scale.Range:Maximum")
                (unwired) 0.0 ("Y Scale.Range:Minimum")
                (unwired) 600.0 ("X Scale.Range:Maximum")
                (unwired) 0.0 ("X Scale.Range:Minimum")
              }
            }
          }
          frame #4 {
            n899 = case shown="True" "RSTCOF 3" {
              frame False {
              }
              frame True {
                n900 = property on="Electronic contact resistance ( % )" class="WFChart (strict)"("XScale.Minimum"=0.0 ("X Scale.Range:Minimum"), "XScale.Maximum"=600.0 ("X Scale.Range:Maximum"), "YScale.Minimum"=0.0 ("Y Scale.Range:Minimum"), "YScale.Maximum"=100.0 ("Y Scale.Range:Maximum")) -> ()  [unwired: 2 in, 2 out]
              }
            }
          }
        }
        n901 = case shown="True" "Case Constant\n(See Context Help) 13" {
          frame False {
          }
          frame True {
            w1948 = TRUE ("Heater")
            n902 = local write "Humidity"(w1948) -> ()
            n903 = local write "Heater Button"(w1948) -> ()
            n904 = local read "TEST STANDARD"() -> (w1951:T2)
            n905 = local read "TEST STANDARD"() -> (w1946:T2)
            n906 = Equal?(x=w1951, y=enum16{"ASTM D6079", "ISO 12156", "Custom"}."ISO 12156" ("Test Standard")) -> (x = y?=w1949:bool)
            n907 = Equal?(x=w1946, y=enum16{"ASTM D6079", "ISO 12156", "Custom"}."ASTM D6079" ("Test Standard")) -> (x = y?=w1945:bool)
            n908 = case shown="True" w1949 {
              frame False {
              }
              frame True {
                n909 = local write "airtempflg"(FALSE ("airtempflg")) -> ()
                n910 = local write "Heater"(TRUE ("Heater")) -> ()
              }
            }
            n911 = case shown="True" w1945 {
              frame False {
              }
              frame True {
                n912 = local write "airtempflg"(TRUE ("airtempflg")) -> ()
                n913 = local write "Heater"(FALSE ("Heater")) -> ()
              }
            }
          }
        }
        n914 = local read "RUN"() -> (w1892:bool)
        n915 = case shown="True" w1892 {
          tunnel: [FALSE ("TEST RUNNING") TRUE ("TEST RUNNING")] -> w1883
          frame False {
            w2022 = 0.0 ("Flag")
            n916 = local write "Flag"(w2022) -> ()
            n917 = local write "Time Remaining"(w2022) -> ()
            n918 = local write "Elapsed time"(0.0 ("elapsedtime")) -> ()
          }
          frame True {
            n919 = local write "Flag"(10.0 ("Flag")) -> ()
          }
        }
        n920 = local read "Flag"() -> (w1889:dbl)
        n921 = local read "RUN"() -> (w1886:bool)
        n922 = Equal?(x=w1889, y=10.0) -> (x = y?=w1887:bool)
        n923 = Not(x=w1886) -> (.not. x?=w1885:bool)
        n924 = And(x=w1887, y=w1885) -> (x .and. y?=w1884:bool)
        n925 = case shown="True" w1884 {
          frame False {
          }
          frame True {
            w1999 = FALSE ("Heater Button")
            n926 = local write "Heater Button"(w1999) -> ()
            n927 = local write "Humidity"(w1999) -> ()
          }
        }
        n928 = local write "Save"(w1883) -> ()
        n929 = local write "Test \nStatus"(w1883) -> ()
        n930 = local write "st enable"(w1883) -> ()
        n931 = local write "PWR"(w1883) -> ()
        n932 = local read "Set Temp"() -> (w1845:dbl)
        n933 = local read "SetTemp"() -> (w1847:dbl)
        n934 = local read "Set Rh"() -> (w1846:dbl)
        n935 = local read "Amb temp"() -> (w1844:dbl)
        n936 = local read "Humidity ( Rh )"() -> (w1843:dbl)
        n937 = local read "TEMP"() -> (w1842:dbl)
        n938 = Add(x=w1847, y=w1872) -> (x+y=w1873:dbl)
        n939 = Subtract(x=w1847, y=w1872) -> (x-y=w1874:dbl)
        n940 = Add(x=w1846, y=w1871) -> (x+y=w1870:dbl)
        n941 = Subtract(x=w1846, y=w1871) -> (x-y=w1869:dbl)
        n942 = Add(x=w1845, y=w1866) -> (x+y=w1867:dbl)
        n943 = Subtract(x=w1845, y=w1866) -> (x-y=w1868:dbl)
        n944 = In Range and Coerce(upper limit=w1873, x=w1844, lower limit=w1874) -> (In Range?=w1863:bool)  [unwired: 1 out]
        n945 = In Range and Coerce(upper limit=w1870, x=w1843, lower limit=w1869) -> (In Range?=w1861:bool)  [unwired: 1 out]
        n946 = In Range and Coerce(upper limit=w1867, x=w1842, lower limit=w1868) -> (In Range?=w1859:bool)  [unwired: 1 out]
        n947 = case shown="True" w1863 {
          tunnel: [FALSE ("RUN") TRUE ("RUN")] -> w1862
          tunnel: [_ 1] -> w1855
          frame False {
          }
          frame True {
          }
        }
        n948 = case shown="True" w1861 {
          tunnel: [FALSE ("RUN") TRUE ("RUN")] -> w1860
          tunnel: [_ 2] -> w1854
          frame False {
          }
          frame True {
          }
        }
        n949 = case shown="True" w1859 {
          tunnel: [FALSE ("RUN") TRUE ("RUN")] -> w1858
          tunnel: [_ 3] -> w1853
          frame False {
          }
          frame True {
          }
        }
        n950 = local read "airtempflg"() -> (w1864:bool)
        n951 = Or(x=w1864, y=w1862) -> (x .or. y?=w1865:bool)
        n952 = Build Array(w1855, w1854, w1853) -> (w1851:i32[])
        n953 = Compound Arithmetic op=AND(w1865, w1860, w1858) -> ()  [unwired: 1 out]
        n954 = case shown="True" "Case Constant\n(See Context Help) 14" {
          frame False {
          }
          frame True {
            w1942 = FALSE ("autostrtflg")
            n955 = local write "autostrtflg"(w1942) -> ()
            n956 = local write "autostart"(w1942) -> ()
            n957 = local write "RUN"(TRUE ("RUN")) -> ()
            n958 = local write "String 14"(" Running....." ("String 14")) -> ()
          }
        }
        n959 = Insert Into Array(array=string[] ["Air Temperature has reached set value,", "Humidity has reached set value,", "Sample Temperaturehas reached set value,", ""], index=0, new element="") -> (w1850:string[])
        n960 = for {
          tunnel: w1851 -> [w1932] mode=indexing
          tunnel: w1850 -> [w1931]
          shift-right: [w1928] -> w1849
          shift-left: "" -> [w1930]
          n961 = Index Array(array=w1931, index=w1932) -> (element=w1929:string)
          n962 = Concatenate Strings(w1929, w1930) -> (w1928:string)
        }
        n963 = local write "autostart 2"(w1849) -> ()
      }
      frame 1 {
        # "Elapsed time\ncof\nstroke\nAir temp\nTemp\nHumidity"
        n964 = case shown="True" "OPEN 4" {
          frame False {
          }
          frame True {
            (unwired) 0  # existing file
            w2452 = "Choose a datalog file to open"  # prompt
            n965 = local write "OPEN 4"(FALSE ("OPEN 1")) -> ()
            n966 = String To Path(string="C:\\LAB-IQ-NXT\\Data\\") -> (path=w2437:path)
